vi "P3 E1 RLJ 2015640305.vi"() -> ()   [LabVIEW 2016]
doc: "Use this template to build a simple state machine design pattern. Each state executes code and determines which state to transition to."
uses:
  State.ctl
  Data.ctl
  Control 3.ctl
panel:
  in  "abortar":bool
  in  "Exit":bool
  out "Tab":T1(tab)
  in  "id":bool
  out "Boolean":bool
  out "Pict Ring":i32(ring)
  in  "ok":bool
  in  "0":bool
  in  "8":bool
  in  "9":bool
  in  "7":bool
  in  "6":bool
  in  "5":bool
  in  "4":bool
  in  "3":bool
  in  "2":bool
  in  "1":bool
  out "concatenated string 2":string
  in  "s 2":bool
  out "String 3":string
  in  "edo de cuenta":bool
  in  "deposito oc":bool
  in  "donativo":bool
  in  "pago de tiempo aire":bool
  in  "pago de tarjeta":bool
  in  "retiro":bool
  in  "SALIR":bool
  in  "ingresar":bool
  out "String":string
  in  "Numeric Control 2":dbl
  in  "abonar":bool
  in  "Numeric Control":dbl
  out "String 2":string
  out "Array 2":bool[](array[boolean])
  in  "100":bool
  in  "200":bool
  in  "300":bool
  in  "500":bool
  out "String 4":string
  in  "CDH Tepeyac":bool
  in  "CILAS":bool
  in  "ALAMPYME":bool
  in  "nicolasa":bool
  out "String 6":string
  in  "pedro":bool
  in  "juan":bool
  in  "s 3":bool
  out "concate":string
  in  "ok 2":bool
  in  "0 2":bool
  in  "8 2":bool
  in  "9 2":bool
  in  "7 2":bool
  in  "6 2":bool
  in  "5 2":bool
  in  "4 2":bool
  in  "3 2":bool
  in  "2 2":bool
  in  "1 2":bool
  out "String 7":string
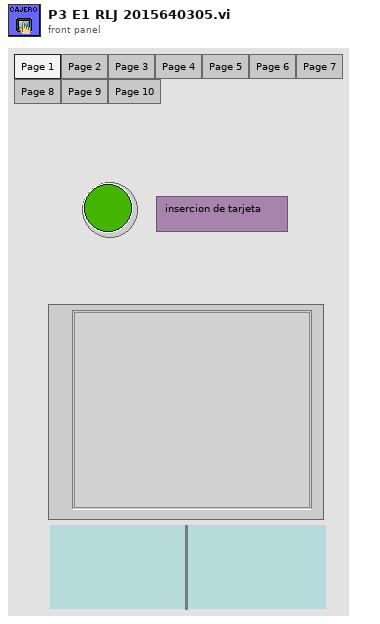
[diagram p1: front panel]
types:
  T1 = enum32{"Page 1", "Page 2", "Page 3", "Page 4", "Page 5", "Page 6", "Page 7", "Page 8", "Page 9", "Page 10"}
  T2 = typedef "Data.ctl" = cluster{"true/false":bool, "String 1":string, "saldo":dbl, "deuda":dbl, "id":bool, "pag1":bool, "seleccion":bool, "edo de cuentas":string, "cuenta error":dbl}
  T3 = typedef "State.ctl" = enum16{"Initialize", "Wait for Event", "id", "contraseña", "error", "retiro de efectivo", "pago de tarjeta", "compra de tiempo aire", "estado de cuenta", "donativo", "deposito a otra cuentas", "teclado", "menu", "abortar", "Exit"}
  T4 = typedef "Control 3.ctl" = enum32{"Page 1", "Page 2", "Page 3", "Page 4", "Page 5", "Page 6", "Page 7", "Page 8", "Page 9", "Page 10"}
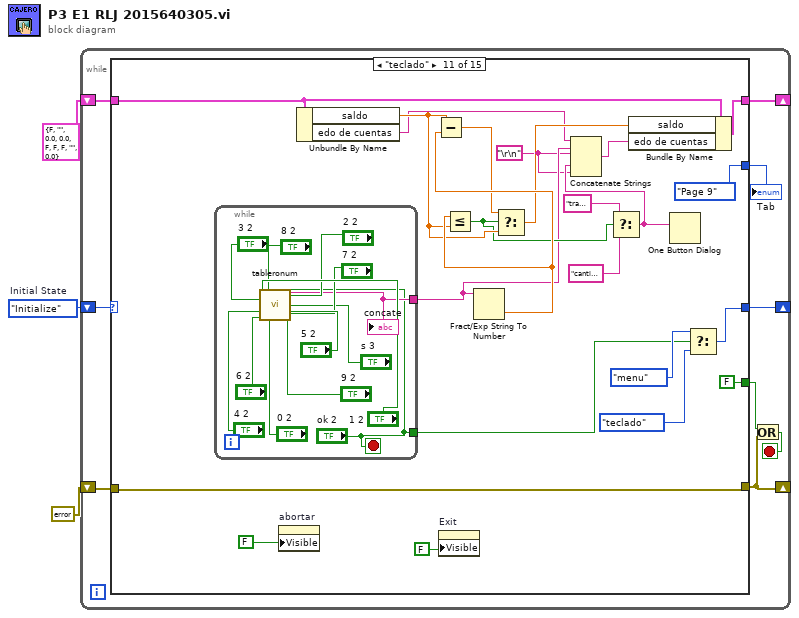
[diagram p0: block diagram]
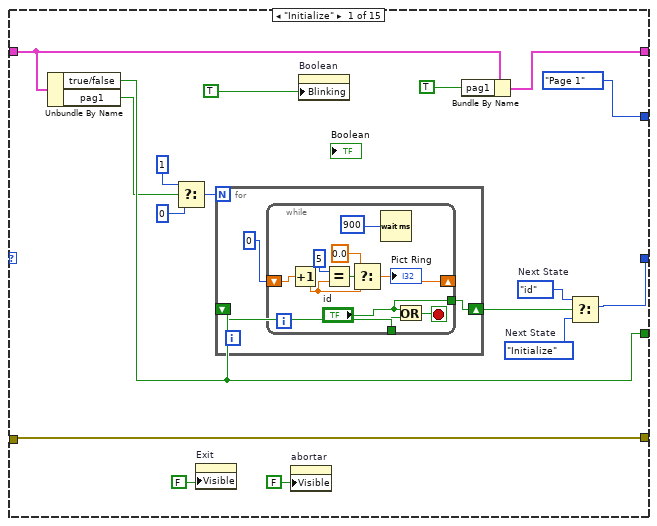
[diagram p2: hidden frame]
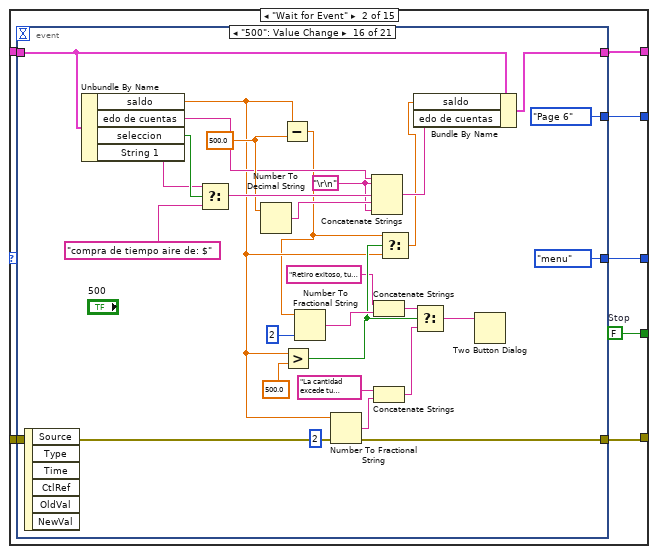
[diagram p3: hidden frame]
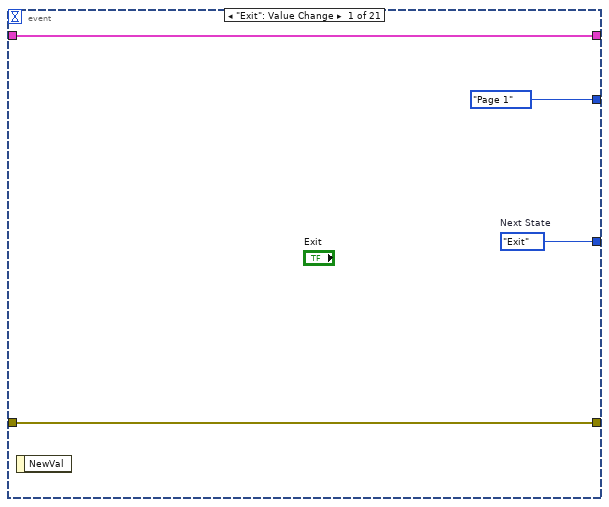
[diagram p4: hidden frame]
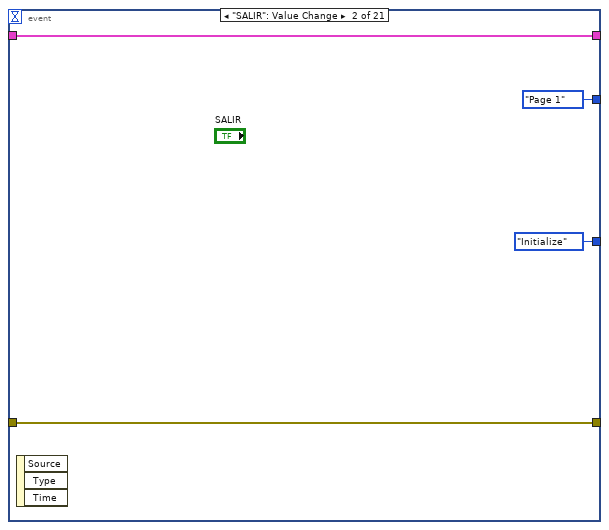
[diagram p5: hidden frame]
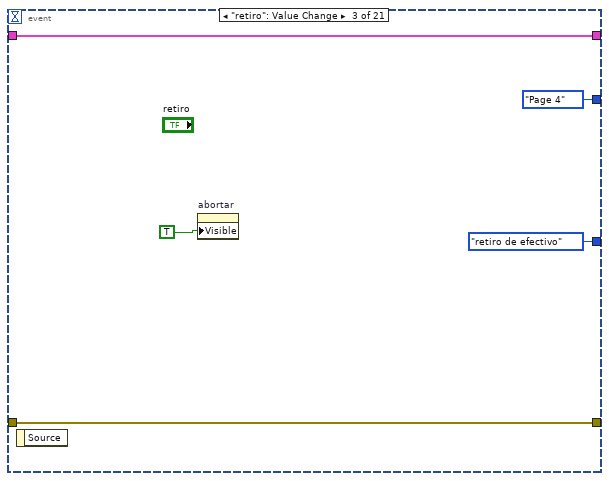
[diagram p6: hidden frame]
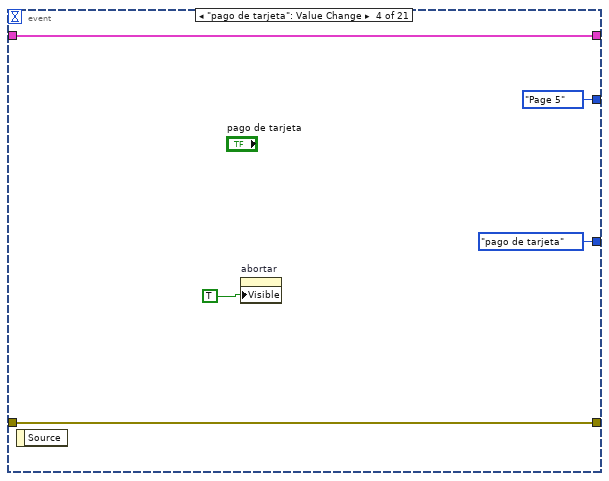
[diagram p7: hidden frame]
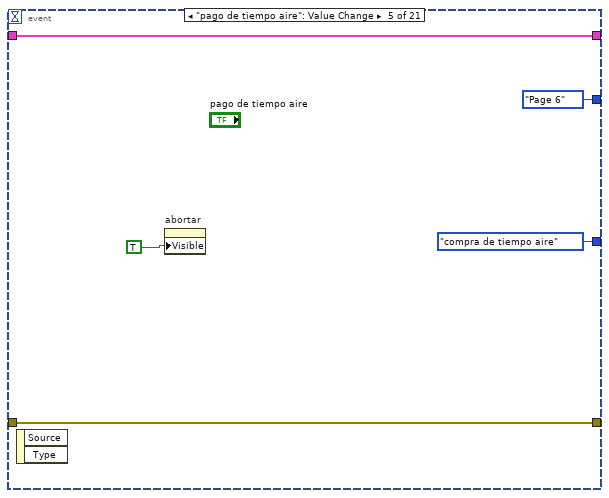
[diagram p8: hidden frame]
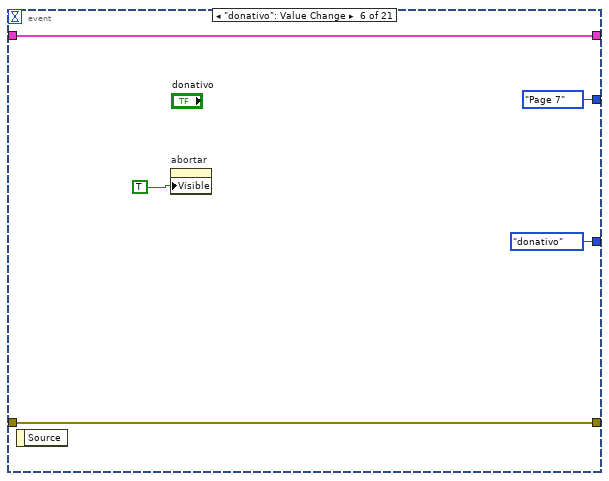
[diagram p9: hidden frame]
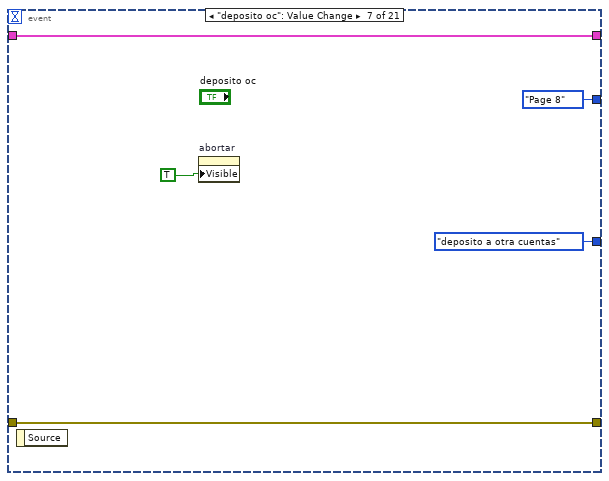
[diagram p10: hidden frame]
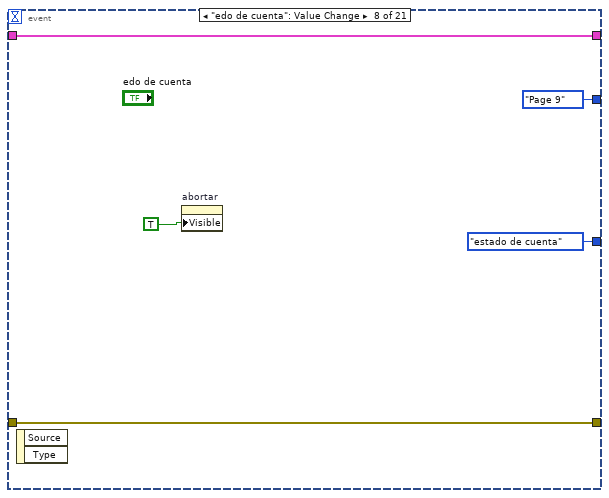
[diagram p11: hidden frame]
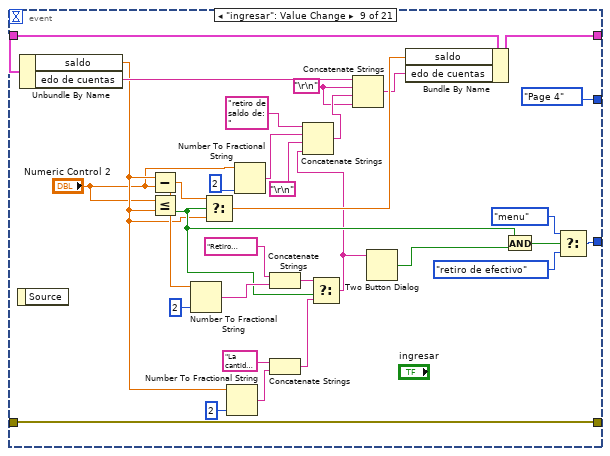
[diagram p12: hidden frame]
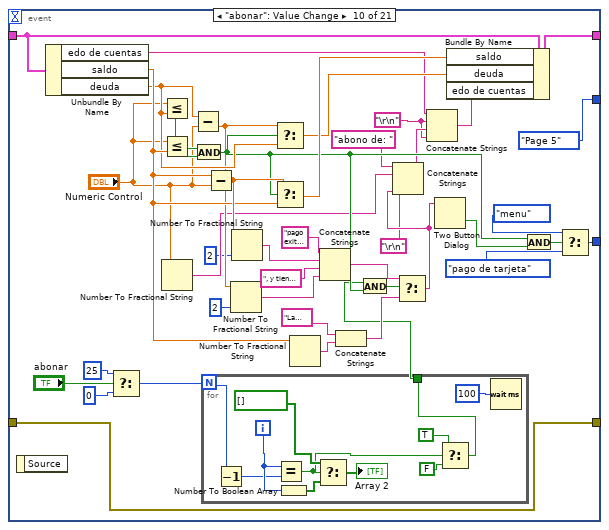
[diagram p13: hidden frame]
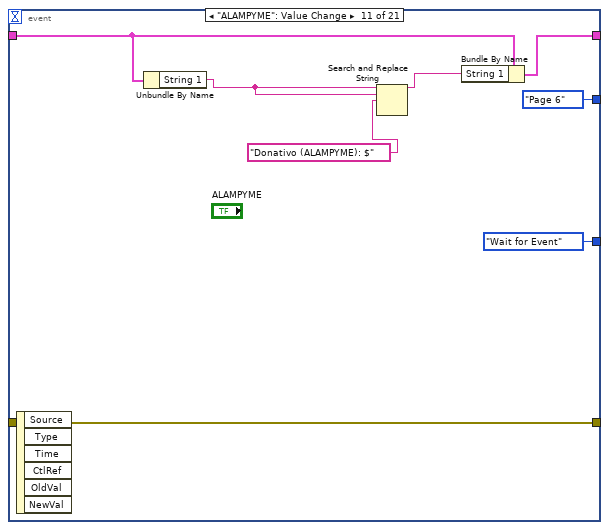
[diagram p14: hidden frame]
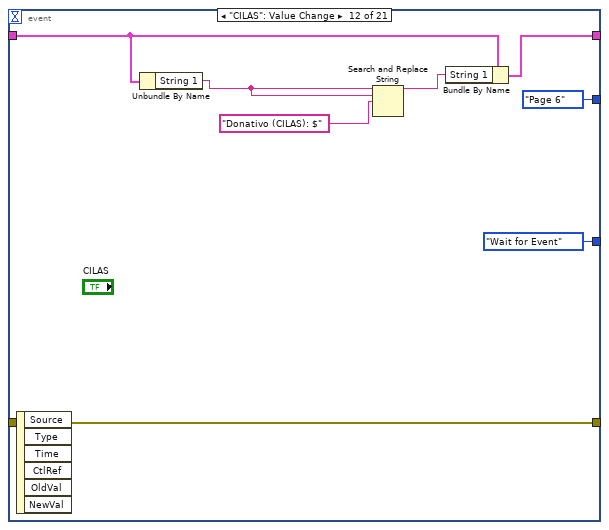
[diagram p15: hidden frame]
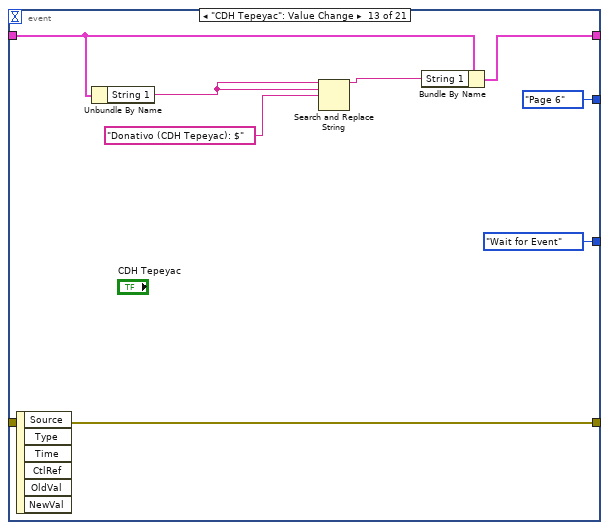
[diagram p16: hidden frame]
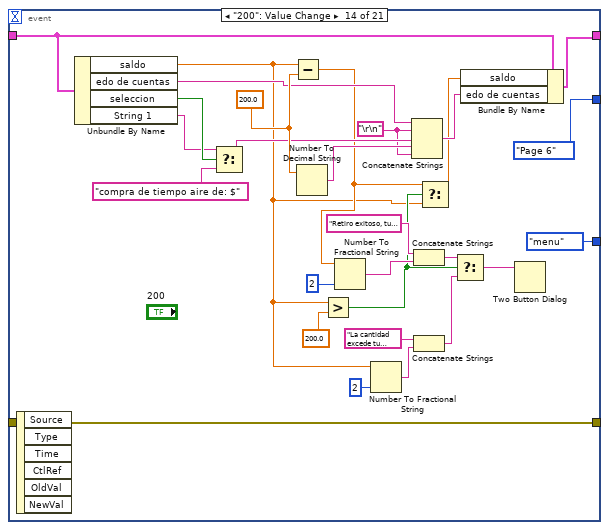
[diagram p17: hidden frame]
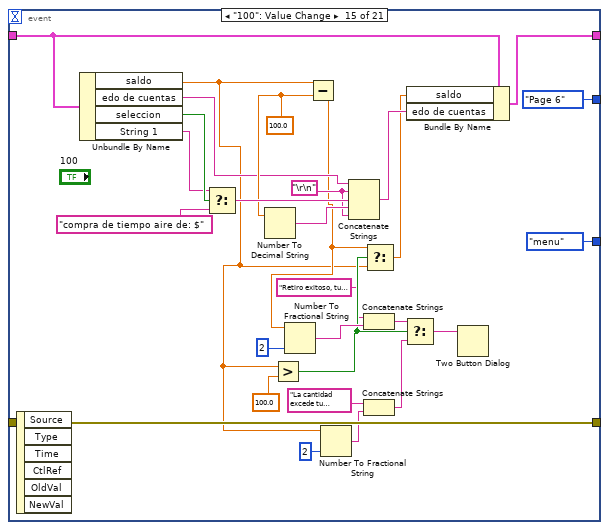
[diagram p18: hidden frame]
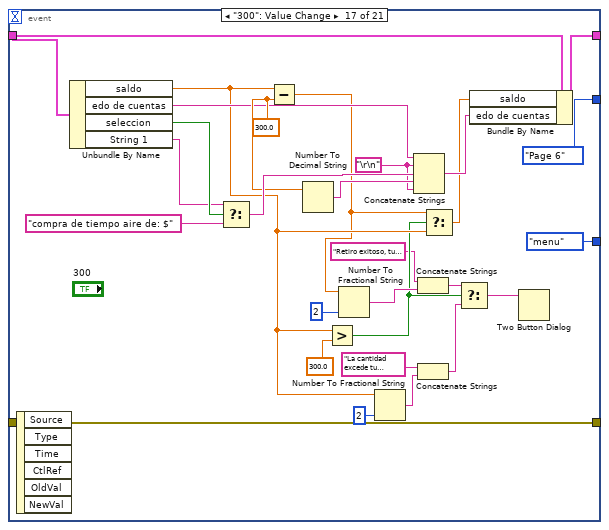
[diagram p19: hidden frame]
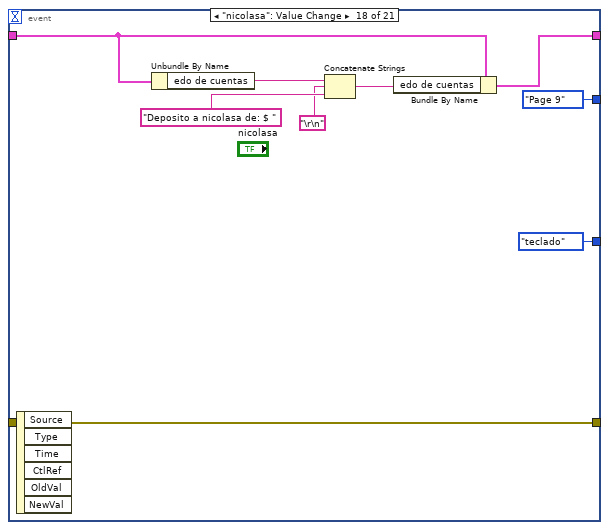
[diagram p20: hidden frame]
diagram:
  w1 = State."Initialize"  # Initial State
  n1 = while {
    shift-right: [w11] -> _
    shift-left: w1 -> [w12]
    shift-right: [w6] -> _
    shift-left: T2 {"true/false"=FALSE, "String 1"="", "saldo"=0.0, "deuda"=0.0, "id"=FALSE, "pag1"=FALSE, "seleccion"=FALSE, "edo de cuentas"="", "cuenta error"=0.0} ("Data") -> [w10]
    shift-right: [w4] -> _
    shift-left: errorcluster {"status"=FALSE, "code"=0, "source"=""} ("error constant") -> [w9]
    stop <- w8 stop-if-true
    # "Main VI State Machine"
    n2 = case shown="\"teclado\"" w12 {
      tunnel: [w28 w49 w344 w373 w393 State."Wait for Event" ("(Value Not Used)") State."Wait for Event" ("(Value Not Used)") State."Wait for Event" ("(Value Not Used)") State."Wait for Event" ("(Value Not Used)") State."Wait for Event" ("(Value Not Used)") w484 State."Wait for Event" ("(Value Not Used)") State."Wait for Event" ("(Value Not Used)") State."menu" ("(Value Not Used)") State."Initialize" ("(Value Not Used)")] -> w11
      tunnel: [w22 w48 FALSE ("Stop Loop?") FALSE ("Stop Loop?") FALSE ("Stop Loop?") FALSE ("Stop Loop?") FALSE ("Stop Loop?") FALSE ("Stop Loop?") FALSE ("Stop Loop?") FALSE ("Stop Loop?") FALSE ("Stop Loop?") FALSE ("Stop Loop?") FALSE ("Stop Loop?") FALSE ("Stop Loop?") TRUE ("Stop Loop?")] -> w5
      tunnel: w10 -> [w16 w47 w341 w371 w385 w415 w425 w435 w451 w456 w487 w505 w514 w531 w536]
      tunnel: [w15 w46 w341 w372 w384 w415 w425 w435 w450 w456 w488 w505 w522 w531 w536] -> w6
      tunnel: w9 -> [w29 w45 w349 w379 w398 w418 w429 w447 w455 w468 w491 w512 w526 w530 w535]
      tunnel: [w29 w44 w349 w379 w398 w418 w429 w447 w455 w468 w491 w512 w526 w530 w535] -> w4
      tunnel: [Control_3."Page 1" ("Tab Control") w43 Control_3."Page 2" ("Tab Control") w369 w389 Control_3."Page 3" ("Tab Control") Control_3."Page 4" ("Tab Control") Control_3."Page 5" ("Tab Control") Control_3."Page 6" ("Tab Control") Control_3."Page 8" ("Tab Control") Control_3."Page 9" ("Tab Control") Control_3."Page 10" ("Tab Control") Control_3."Page 7" ("Tab Control") Control_3."Page 3" ("Tab Control") Control_3."Page 1" ("Tab Control")] -> w7
      frame "Initialize" {
        w26 = State."Initialize"  # Next State
        w27 = State."id"  # Next State
        # "Initialize - Initialize the application."
        n3 = Unbundle By Name(w16) -> ("true/false"=w22:bool, "pag1"=w17:bool)
        n4 = Select(t=1, s=w17, f=0) -> (s? t:f=w20:i32)
        n5 = property on="Exit" class="Bool"("Visible"=FALSE) -> ()  [unwired: 2 in, 2 out]
        n6 = for {
          N: w20 -> [_]
          shift-right: [w30] -> w21
          shift-left: w22 -> [w31]
          n7 = while {
            shift-right: [w39] -> _
            shift-left: 0 -> [w41]
            tunnel: w31 -> [w34]
            tunnel: ["id"] -> w30
            stop <- w35 stop-if-true
            n8 = Increment(x=w41) -> (x+1=w36:dbl)
            n9 = Equal?(x=5, y=w36) -> (x = y?=w38:bool)
            n10 = Select(t=0.0, s=w38, f=w36) -> (s? t:f=w39:dbl)
            "Pict Ring" <- w39
            n11 = Wait (ms)(milliseconds to wait=u32 900) -> ()  [unwired: 1 out]
            n12 = Or(x="id", y=w34) -> (x .or. y?=w35:bool)
          }
        }
        n13 = property on="abortar" class="Bool"("Visible"=FALSE) -> ()  [unwired: 2 in, 2 out]
        n14 = property on="Boolean" class="Bool (strict)"("Blinking"=TRUE) -> ()  [unwired: 2 in, 2 out]
        n15 = Bundle By Name(cluster=w16, "pag1"=TRUE ("corrimiento")) -> (w15:T2)
        n16 = Select(t=w27, s=w21, f=w26) -> (s? t:f=w28:T3)
      }
      frame "Wait for Event" {
        w48 = FALSE  # Stop
        n17 = event shown="[15] \"500\": Value Change" {
          selector: _ -> [_ _ _ _ _ _ _ _ _ _ _ _ _ _ _ _ _ _ _ _ _]
          dyn-events: _ -> [_ _ _ _ _ _ _ _ _ _ _ _ _ _ _ _ _ _ _ _ _]
          timeout: _ -> [_ _ _ _ _ _ _ _ _ _ _ _ _ _ _ _ _ _ _ _ _]
          tunnel: [w53 State."Initialize" ("f") State."retiro de efectivo" ("f") State."pago de tarjeta" ("f") State."compra de tiempo aire" ("f") State."donativo" ("f") State."deposito a otra cuentas" ("f") State."estado de cuenta" ("f") w108 w145 State."Wait for Event" ("f") State."Wait for Event" ("f") State."Wait for Event" ("f") State."menu" ("f") State."menu" ("f") State."menu" ("f") State."menu" ("f") State."teclado" ("f") State."teclado" ("f") State."teclado" ("f") State."menu" ("f")] -> w49
          tunnel: w47 -> [w52 w57 w62 w67 w72 w77 w82 w87 w104 w147 w176 w181 w189 w221 w249 w277 w305 w312 w322 w330 w339]
          tunnel: [w52 w57 w62 w67 w72 w77 w82 w87 w101 w146 w179 w187 w195 w220 w248 w276 w304 w311 w323 w329 w339] -> w46
          tunnel: w45 -> [w51 w56 w61 w66 w71 w76 w81 w86 w118 w161 w180 w188 w196 w224 w252 w280 w308 w317 w326 w335 w338]
          tunnel: [w51 w56 w61 w66 w71 w76 w81 w86 w118 w161 w180 w188 w196 w224 w252 w280 w308 w317 w326 w335 w338] -> w44
          tunnel: [Control_3."Page 1" ("Tab Control") Control_3."Page 1" ("Tab Control") Control_3."Page 4" ("Tab Control") Control_3."Page 5" ("Tab Control") Control_3."Page 6" ("Tab Control") Control_3."Page 7" ("Tab Control") Control_3."Page 8" ("Tab Control") Control_3."Page 9" ("Tab Control") Control_3."Page 4" ("Tab Control") Control_3."Page 5" ("Tab Control") Control_3."Page 6" ("Tab Control") Control_3."Page 6" ("Tab Control") Control_3."Page 6" ("Tab Control") Control_3."Page 6" ("Tab Control") Control_3."Page 6" ("Tab Control") Control_3."Page 6" ("Tab Control") Control_3."Page 6" ("Tab Control") Control_3."Page 9" ("Tab Control") Control_3."Page 9" ("Tab Control") Control_3."Page 9" ("Tab Control") Control_3."Page 3" ("Tab Control")] -> w43
          event "Exit": Value Change {
            w53 = State."Exit"  # Next State
            n18 = event-data() -> ()  [unwired: 1 in, 1 out]
          }
          event "SALIR": Value Change {
            n19 = event-data() -> ()  [unwired: 1 in, 3 out]
          }
          event "retiro": Value Change {
            n20 = event-data() -> ()  [unwired: 1 in, 1 out]
            n21 = property on="abortar" class="Bool"("Visible"=TRUE) -> ()  [unwired: 2 in, 2 out]
          }
          event "pago de tarjeta": Value Change {
            n22 = event-data() -> ()  [unwired: 1 in, 1 out]
            n23 = property on="abortar" class="Bool"("Visible"=TRUE) -> ()  [unwired: 2 in, 2 out]
          }
          event "pago de tiempo aire": Value Change {
            n24 = event-data() -> ()  [unwired: 1 in, 2 out]
            n25 = property on="abortar" class="Bool"("Visible"=TRUE) -> ()  [unwired: 2 in, 2 out]
          }
          event "donativo": Value Change {
            n26 = event-data() -> ()  [unwired: 1 in, 1 out]
            n27 = property on="abortar" class="Bool"("Visible"=TRUE) -> ()  [unwired: 2 in, 2 out]
          }
          event "deposito oc": Value Change {
            n28 = event-data() -> ()  [unwired: 1 in, 1 out]
            n29 = property on="abortar" class="Bool"("Visible"=TRUE) -> ()  [unwired: 2 in, 2 out]
          }
          event "edo de cuenta": Value Change {
            n30 = event-data() -> ()  [unwired: 1 in, 2 out]
            n31 = property on="abortar" class="Bool"("Visible"=TRUE) -> ()  [unwired: 2 in, 2 out]
          }
          event "ingresar": Value Change {
            w91 = "\r\n"
            n32 = event-data() -> ()  [unwired: 1 in, 1 out]
            n33 = Unbundle By Name(w104) -> ("saldo"=w93:dbl, "edo de cuentas"=w100:string)
            n34 = Subtract(x=w93, y="Numeric Control 2") -> (x-y=w117:dbl)
            n35 = Less Or Equal?(x="Numeric Control 2", y=w93) -> (x <= y?=w110:bool)
            n36 = Number To Fractional String(number=w117, precision (6)=i16 2) -> (F-format string=w116:string)  [unwired: 2 in]
            n37 = Select(t=w117, s=w110, f=w93) -> (s? t:f=w103:dbl)
            n38 = Number To Fractional String(number=w93, precision (6)=i16 2) -> (F-format string=w113:string)  [unwired: 2 in]
            n39 = Number To Fractional String(number="Numeric Control 2", precision (6)=i16 2) -> (F-format string=w98:string)  [unwired: 2 in]
            n40 = Concatenate Strings("Retiro exitoso, tu saldo actual es de: \n" ("string"), w116) -> (w115:string)
            n41 = Concatenate Strings("La cantidad excede tu credito, el cual es de: \n" ("string"), w113) -> (w112:string)
            n42 = Select(t=w115, s=w110, f=w112) -> (s? t:f=w95:string)
            n43 = Concatenate Strings("retiro de saldo de: " ("string"), w98, "\r\n", w95) -> (w96:string)
            n44 = Concatenate Strings(w100, w91, w96, w91) -> (w99:string)
            n45 = Two Button Dialog(message=w95) -> (T button?=w111:bool)  [unwired: 2 in]
            n46 = Bundle By Name(cluster=w104, "saldo"=w103, "edo de cuentas"=w99) -> (w101:T2)
            n47 = And(x=w110, y=w111) -> (x .and. y?=w109:bool)
            n48 = Select(t=State."menu" ("Next State"), s=w109, f=State."retiro de efectivo") -> (s? t:f=w108:T3)
          }
          event "abonar": Value Change {
            w123 = "\r\n"
            n49 = event-data() -> ()  [unwired: 1 in, 1 out]
            n50 = Unbundle By Name(w147) -> ("edo de cuentas"=w130:string, "saldo"=w154:dbl, "deuda"=w141:dbl)
            n51 = Select(t=25, s="abonar", f=0) -> (s? t:f=w137:i32)
            n52 = Less Or Equal?(x="Numeric Control", y=w141) -> (x <= y?=w144:bool)
            n53 = Less Or Equal?(x="Numeric Control", y=w154) -> (x <= y?=w143:bool)
            n54 = Number To Fractional String(number="Numeric Control") -> (F-format string=w127:string)  [unwired: 3 in]
            n55 = Subtract(x=w141, y="Numeric Control") -> (x-y=w132:dbl)
            n56 = And(x=w144, y=w143) -> (x .and. y?=w136:bool)
            n57 = for {
              N: w137 -> [w170]
              tunnel: [w162] -> w134
              i -> [w171]
              n58 = Decrement(x=w170) -> (x-1=w169:i32)
              n59 = Equal?(x=w171, y=w169) -> (x = y?=w165:bool)
              n60 = Number To Boolean Array(number=w171) -> (Boolean array=w168:bool[])
              n61 = Select(t=bool[] [], s=w165, f=w168) -> (s? t:f=→"Array 2":bool[])
              n62 = Select(t=TRUE, s=w165, f=FALSE) -> (s? t:f=w162:bool)
              n63 = Wait (ms)(milliseconds to wait=u32 100) -> ()  [unwired: 1 out]
            }
            n64 = Subtract(x=w154, y="Numeric Control") -> (x-y=w160:dbl)
            n65 = Number To Fractional String(number=w132, precision (6)=i16 2) -> (F-format string=w122:string)  [unwired: 2 in]
            n66 = Number To Fractional String(number=w160, precision (6)=i16 2) -> (F-format string=w159:string)  [unwired: 2 in]
            n67 = Select(t=w132, s=w136, f=w141) -> (s? t:f=w142:dbl)
            n68 = Select(t=w160, s=w136, f=w154) -> (s? t:f=w148:dbl)
            n69 = Number To Fractional String(number=w154) -> (F-format string=w156:string)  [unwired: 3 in]
            n70 = Concatenate Strings("pago exitoso, tu saldo actual es de: \n" ("string"), w159, ", y tienes un adeudo de: " ("string"), w122) -> (w158:string)
            n71 = Concatenate Strings("La cantidad excede tu credito, el cual es de: \n" ("string"), w156) -> (w155:string)
            n72 = And(x=w134, y=w136) -> (x .and. y?=w133:bool)
            n73 = Select(t=w158, s=w133, f=w155) -> (s? t:f=w125:string)
            n74 = Concatenate Strings("abono de: " ("string"), w127, "\r\n", w125) -> (w126:string)
            n75 = Concatenate Strings(w130, w123, w126, w123) -> (w131:string)
            n76 = Two Button Dialog(message=w125) -> (T button?=w153:bool)  [unwired: 2 in]
            n77 = Bundle By Name(cluster=w147, "saldo"=w148, "deuda"=w142, "edo de cuentas"=w131) -> (w146:T2)
            n78 = And(x=w136, y=w153) -> (x .and. y?=w152:bool)
            n79 = Select(t=State."menu" ("Next State"), s=w152, f=State."pago de tarjeta") -> (s? t:f=w145:T3)
          }
          event "ALAMPYME": Value Change {
            n80 = event-data() -> ()  [unwired: 1 in, 6 out]
            n81 = Unbundle By Name(w176) -> ("String 1"=w175:string)
            n82 = Search and Replace String(input string=w175, search string=w175, replace string="Donativo (ALAMPYME): $" ("String <Replace Me>")) -> (result string=w173:string)  [unwired: 5 in, 3 out]
            n83 = Bundle By Name(cluster=w176, "String 1"=w173) -> (w179:T2)
          }
          event "CILAS": Value Change {
            n84 = event-data() -> ()  [unwired: 1 in, 6 out]
            n85 = Unbundle By Name(w181) -> ("String 1"=w184:string)
            n86 = Search and Replace String(input string=w184, search string=w184, replace string="Donativo (CILAS): $" ("String <Replace Me>")) -> (result string=w183:string)  [unwired: 5 in, 3 out]
            n87 = Bundle By Name(cluster=w181, "String 1"=w183) -> (w187:T2)
          }
          event "CDH Tepeyac": Value Change {
            n88 = event-data() -> ()  [unwired: 1 in, 6 out]
            n89 = Unbundle By Name(w189) -> ("String 1"=w192:string)
            n90 = Search and Replace String(input string=w192, search string=w192, replace string="Donativo (CDH Tepeyac): $" ("String <Replace Me>")) -> (result string=w190:string)  [unwired: 5 in, 3 out]
            n91 = Bundle By Name(cluster=w189, "String 1"=w190) -> (w195:T2)
          }
          event "200": Value Change {
            w211 = "\r\n"
            w219 = 200.0 ("y")
            n92 = event-data() -> ()  [unwired: 1 in, 6 out]
            n93 = Unbundle By Name(w221) -> ("saldo"=w198:dbl, "edo de cuentas"=w212:string, "seleccion"=w217:bool, "String 1"=w213:string)
            n94 = Select(t=w213, s=w217, f="compra de tiempo aire de: $") -> (s? t:f=w215:string)
            n95 = Subtract(x=w198, y=w219) -> (x-y=w199:dbl)
            n96 = Number To Decimal String(number=w219) -> (decimal integer string=w214:string)  [unwired: 1 in]
            n97 = Greater?(x=w198, y=200.0) -> (0:w200:bool)
            n98 = Number To Fractional String(number=w199, precision (6)=i16 2) -> (F-format string=w210:string)  [unwired: 2 in]
            n99 = Number To Fractional String(number=w198, precision (6)=i16 2) -> (F-format string=w207:string)  [unwired: 2 in]
            n100 = Concatenate Strings(w212, w211, w215, w214, w211) -> (w218:string)
            n101 = Concatenate Strings("Retiro exitoso, tu saldo actual es de: \n" ("string"), w210) -> (w209:string)
            n102 = Concatenate Strings("La cantidad excede tu credito, el cual es de: \n" ("string"), w207) -> (w206:string)
            n103 = Select(t=w199, s=w200, f=w198) -> (s? t:f=w197:dbl)
            n104 = Select(t=w209, s=w200, f=w206) -> (s? t:f=w203:string)
            n105 = Bundle By Name(cluster=w221, "saldo"=w197, "edo de cuentas"=w218) -> (w220:T2)
            n106 = Two Button Dialog(message=w203) -> ()  [unwired: 2 in, 1 out]
          }
          event "100": Value Change {
            w239 = "\r\n"
            w243 = 100.0 ("y")
            n107 = event-data() -> ()  [unwired: 1 in, 6 out]
            n108 = Unbundle By Name(w249) -> ("saldo"=w226:dbl, "edo de cuentas"=w240:string, "seleccion"=w242:bool, "String 1"=w241:string)
            n109 = Select(t=w241, s=w242, f="compra de tiempo aire de: $") -> (s? t:f=w246:string)
            n110 = Number To Decimal String(number=w243) -> (decimal integer string=w245:string)  [unwired: 1 in]
            n111 = Greater?(x=w226, y=100.0) -> (0:w229:bool)
            n112 = Subtract(x=w226, y=w243) -> (x-y=w227:dbl)
            n113 = Number To Fractional String(number=w227, precision (6)=i16 2) -> (F-format string=w238:string)  [unwired: 2 in]
            n114 = Number To Fractional String(number=w226, precision (6)=i16 2) -> (F-format string=w235:string)  [unwired: 2 in]
            n115 = Concatenate Strings(w240, w239, w246, w245, w239) -> (w244:string)
            n116 = Concatenate Strings("Retiro exitoso, tu saldo actual es de: \n" ("string"), w238) -> (w237:string)
            n117 = Concatenate Strings("La cantidad excede tu credito, el cual es de: \n" ("string"), w235) -> (w234:string)
            n118 = Select(t=w227, s=w229, f=w226) -> (s? t:f=w225:dbl)
            n119 = Select(t=w237, s=w229, f=w234) -> (s? t:f=w232:string)
            n120 = Bundle By Name(cluster=w249, "saldo"=w225, "edo de cuentas"=w244) -> (w248:T2)
            n121 = Two Button Dialog(message=w232) -> ()  [unwired: 2 in, 1 out]
          }
          event "500": Value Change {
            w270 = 500.0 ("y")
            w267 = "\r\n"
            n122 = event-data() -> ()  [unwired: 1 in, 6 out]
            n123 = Unbundle By Name(w277) -> ("saldo"=w256:dbl, "edo de cuentas"=w268:string, "seleccion"=w271:bool, "String 1"=w269:string)
            n124 = Select(t=w269, s=w271, f="compra de tiempo aire de: $") -> (s? t:f=w274:string)
            n125 = Number To Decimal String(number=w270) -> (decimal integer string=w273:string)  [unwired: 1 in]
            n126 = Subtract(x=w256, y=w270) -> (x-y=w255:dbl)
            n127 = Greater?(x=w256, y=500.0) -> (0:w257:bool)
            n128 = Number To Fractional String(number=w255, precision (6)=i16 2) -> (F-format string=w266:string)  [unwired: 2 in]
            n129 = Number To Fractional String(number=w256, precision (6)=i16 2) -> (F-format string=w263:string)  [unwired: 2 in]
            n130 = Concatenate Strings(w268, w267, w274, w273, w267) -> (w272:string)
            n131 = Concatenate Strings("Retiro exitoso, tu saldo actual es de: \n" ("string"), w266) -> (w265:string)
            n132 = Concatenate Strings("La cantidad excede tu credito, el cual es de: \n" ("string"), w263) -> (w262:string)
            n133 = Select(t=w255, s=w257, f=w256) -> (s? t:f=w254:dbl)
            n134 = Bundle By Name(cluster=w277, "saldo"=w254, "edo de cuentas"=w272) -> (w276:T2)
            n135 = Select(t=w265, s=w257, f=w262) -> (s? t:f=w260:string)
            n136 = Two Button Dialog(message=w260) -> ()  [unwired: 2 in, 1 out]
          }
          event "300": Value Change {
            w295 = "\r\n"
            w300 = 300.0 ("y")
            n137 = event-data() -> ()  [unwired: 1 in, 6 out]
            n138 = Unbundle By Name(w305) -> ("saldo"=w285:dbl, "edo de cuentas"=w296:string, "seleccion"=w298:bool, "String 1"=w297:string)
            n139 = Select(t=w297, s=w298, f="compra de tiempo aire de: $") -> (s? t:f=w302:string)
            n140 = Subtract(x=w285, y=w300) -> (x-y=w283:dbl)
            n141 = Number To Decimal String(number=w300) -> (decimal integer string=w301:string)  [unwired: 1 in]
            n142 = Greater?(x=w285, y=300.0) -> (0:w284:bool)
            n143 = Number To Fractional String(number=w283, precision (6)=i16 2) -> (F-format string=w294:string)  [unwired: 2 in]
            n144 = Number To Fractional String(number=w285, precision (6)=i16 2) -> (F-format string=w291:string)  [unwired: 2 in]
            n145 = Concatenate Strings(w296, w295, w302, w301, w295) -> (w299:string)
            n146 = Concatenate Strings("Retiro exitoso, tu saldo actual es de: \n" ("string"), w294) -> (w293:string)
            n147 = Concatenate Strings("La cantidad excede tu credito, el cual es de: \n" ("string"), w291) -> (w290:string)
            n148 = Select(t=w283, s=w284, f=w285) -> (s? t:f=w282:dbl)
            n149 = Select(t=w293, s=w284, f=w290) -> (s? t:f=w288:string)
            n150 = Bundle By Name(cluster=w305, "saldo"=w282, "edo de cuentas"=w299) -> (w304:T2)
            n151 = Two Button Dialog(message=w288) -> ()  [unwired: 2 in, 1 out]
          }
          event "nicolasa": Value Change {
            n152 = event-data() -> ()  [unwired: 1 in, 6 out]
            n153 = Unbundle By Name(w312) -> ("edo de cuentas"=w313:string)
            n154 = Concatenate Strings(w313, "\r\n", "Deposito a nicolasa de: $ " ("string")) -> (w314:string)
            n155 = Bundle By Name(cluster=w312, "edo de cuentas"=w314) -> (w311:T2)
          }
          event "juan": Value Change {
            n156 = event-data() -> ()  [unwired: 1 in, 6 out]
            n157 = Unbundle By Name(w322) -> ("edo de cuentas"=w321:string)
            n158 = Concatenate Strings(w321, "\r\n", "Deposito a juan de: $ " ("string")) -> (w320:string)
            n159 = Bundle By Name(cluster=w322, "edo de cuentas"=w320) -> (w323:T2)
          }
          event "pedro": Value Change {
            n160 = event-data() -> ()  [unwired: 1 in, 6 out]
            n161 = Unbundle By Name(w330) -> ("edo de cuentas"=w331:string)
            n162 = Concatenate Strings(w331, "\r\n", "Deposito a pedro de: $ " ("string")) -> (w332:string)
            n163 = Bundle By Name(cluster=w330, "edo de cuentas"=w332) -> (w329:T2)
          }
          event "abortar": Value Change {
            n164 = event-data() -> ()  [unwired: 1 in, 2 out]
          }
        }
      }
      frame "contraseña" {
        w345 = State."error"  # Next State
        w346 = State."menu"  # Next State
        n165 = while {
          tunnel: [w352] -> w342
          stop <- "ok" stop-if-true
          n166 = call "tableronum.vi"("1"="1", "8"="8", "OK"="ok", "3"="3", "2"="2", "s 2"="s 2", "4"="4", "5"="5", "6"="6", "0"="0", "7"="7", "9"="9") -> ("concatenated string"=w352:string)  [unwired: 3 in]
          "concatenated string 2" <- w352
        }
        n167 = Unbundle By Name(w341) -> ()  [unwired: 1 out]
        n168 = Equal?(x=w342, y="1393") -> (x = y?=w343:bool)
        n169 = Select(t=w346, s=w343, f=w345) -> (s? t:f=w344:T3)
      }
      frame "error" {
        n170 = Unbundle By Name(w371) -> ("cuenta error"=w370:dbl)
        n171 = Increment(x=w370) -> (x+1=w377:dbl)
        n172 = Equal?(x=w377, y=3.0) -> (x = y?=w366:bool)
        n173 = Bundle By Name(cluster=w371, "cuenta error"=w377, "true/false"=w366) -> (w372:T2)
        n174 = Select(t="Cancelación de sesión" ("message"), s=w366, f="error" ("message")) -> (s? t:f=w363:string)
        n175 = One Button Dialog(message=w363) -> ()  [unwired: 1 in, 1 out]
        n176 = Select(t=Control_3."Page 1" ("Tab Control"), s=w366, f=Control_3."Page 2" ("Tab Control")) -> (s? t:f=w369:T4)
        n177 = Select(t=State."Initialize" ("(Value Not Used)"), s=w366, f=State."contraseña" ("(Value Not Used)")) -> (s? t:f=w373:T3)
      }
      frame "id" {
        w394 = State."Initialize"  # Initial State
        w395 = State."contraseña"  # Initial State
        # "User State 1 - Replace this state with functionality for your own application."
        n178 = Random Number (0-1)() -> (number: 0 to 1=w386:dbl)
        n179 = Random Number (0-1)() -> (number: 0 to 1=w387:dbl)
        n180 = expression code="6000-(1000*x)"(w386) -> (w383:dbl)
        n181 = expression code="10000-(6000*x)"(w387) -> (w381:dbl)
        n182 = To Quad Integer(1:w383) -> (0:w382:i64)
        n183 = To Quad Integer(1:w381) -> (0:w380:i64)
        n184 = Bundle By Name(cluster=w385, "saldo"=w382, "deuda"=w380) -> (w384:T2)
        n185 = Two Button Dialog(message="es usted Ramirez lopez jesus alberto\ncon numero de boleta 2015640305" ("Running User State 1"), 1:"no" ("F button name (\"Cancel\")"), 2:"si" ("T button name (\"OK\")")) -> (T button?=w391:bool)
        n186 = Select(t=w395, s=w391, f=w394) -> (s? t:f=w393:T3)
        n187 = Select(t=Control_3."Page 2" ("Tab Control"), s=w391, f=Control_3."Page 1" ("Tab Control")) -> (s? t:f=w389:T4)
      }
      frame "menu" {
        n188 = Unbundle By Name(w415) -> ("saldo"=w408:dbl, "deuda"=w402:dbl)
        n189 = property on="Exit" class="Bool"("Visible"=TRUE) -> ()  [unwired: 2 in, 2 out]
        n190 = property on="abortar" class="Bool"("Visible"=FALSE) -> ()  [unwired: 2 in, 2 out]
        n191 = Number To Fractional String(number=w402, precision (6)=i16 2) -> (F-format string=w406:string)  [unwired: 2 in]
        n192 = Number To Fractional String(number=w408, precision (6)=i16 2) -> (F-format string=w413:string)  [unwired: 2 in]
        n193 = Concatenate Strings("TU SALDO ES DE:   " ("message"), w413) -> (w410:string)
        n194 = Concatenate Strings("TU DEUDA ES DE:   " ("message"), w406) -> (w409:string)
        n195 = Concatenate Strings(w410, "\r\n", w409) -> (→"String 3":string)
      }
      frame "retiro de efectivo" {
        n196 = Unbundle By Name(w425) -> ("saldo"=w420:dbl)
        n197 = Number To Fractional String(number=w420, precision (6)=i16 2) -> (F-format string=w424:string)  [unwired: 2 in]
        n198 = Concatenate Strings("RETIRO DE EFECTIVO:    \n tu credito es de: " ("string"), w424, "\nIngresa el valor a retirar" ("string")) -> (→"String":string)
      }
      frame "pago de tarjeta" {
        n199 = Unbundle By Name(w435) -> ("saldo"=w440:dbl)
        n200 = Unbundle By Name(w435) -> ("deuda"=w436:dbl)
        n201 = Number To Fractional String(number=w440, precision (6)=i16 2) -> (F-format string=w443:string)  [unwired: 2 in]
        n202 = Number To Fractional String(number=w436, precision (6)=i16 2) -> (F-format string=w439:string)  [unwired: 2 in]
        n203 = Concatenate Strings("PAGO DE TARJETA:    \n tu credito es de: " ("string"), w443, "\nIngresa el valor a retirar" ("string")) -> (w434:string)
        n204 = Concatenate Strings("\nsu adeudo de tarjeta de credito es de: " ("string"), w439, "\nIngresa el valor a abonar" ("string")) -> (w433:string)
        n205 = Concatenate Strings(w434, w433) -> (→"String 2":string)
      }
      frame "compra de tiempo aire" {
        n206 = Bundle By Name(cluster=w451, "String 1"="COMPRA DE TIEMPO AIRE\nselecciona el valor de tu recarga" ("String <Replace Me>"), "seleccion"=FALSE) -> (w450:T2)
      }
      frame "deposito a otra cuentas" {
        w457 = "\r\n"
        n207 = Unbundle By Name(w456) -> ("saldo"=w463:dbl)
        n208 = Number To Fractional String(number=w463, precision (6)=i16 2) -> (F-format string=w460:string)  [unwired: 2 in]
        n209 = Concatenate Strings("DEPOSITO A OTRAS CUENTAS" ("string"), w457, "Tu saldo es de: " ("string"), w457, w460, w457, "Selecciona la persona a la que realizaras el deposito:") -> (→"String 6":string)
      }
      frame "teclado" {
        w472 = "\r\n"
        n210 = while {
          tunnel: [w494] -> w474
          tunnel: ["ok 2"] -> w483
          stop <- "ok 2" stop-if-true
          n211 = call "tableronum.vi"("1"="1 2", "8"="8 2", "OK"="ok 2", "3"="3 2", "2"="2 2", "s 2"="s 3", "4"="4 2", "5"="5 2", "6"="6 2", "0"="0 2", "7"="7 2", "9"="9 2") -> ("concatenated string"=w494:string)  [unwired: 3 in]
          "concate" <- w494
        }
        n212 = property on="abortar" class="Bool"("Visible"=FALSE) -> ()  [unwired: 2 in, 2 out]
        n213 = Unbundle By Name(w487) -> ("saldo"=w479:dbl, "edo de cuentas"=w475:string)
        n214 = property on="Exit" class="Bool"("Visible"=FALSE) -> ()  [unwired: 2 in, 2 out]
        n215 = Fract/Exp String To Number(string=w474) -> (number=w482:dbl)  [unwired: 3 in, 1 out]
        n216 = Subtract(x=w479, y=w482) -> (x-y=w480:dbl)
        n217 = Less Or Equal?(x=w482, y=w479) -> (x <= y?=w478:bool)
        n218 = Select(t=w480, s=w478, f=w479) -> (s? t:f=w481:dbl)
        n219 = Select(t="transaccion exitosa", s=w478, f="cantidad incorrecta") -> (s? t:f=w473:string)
        n220 = Concatenate Strings(w475, w474, w472, w473, w472) -> (w471:string)
        n221 = Bundle By Name(cluster=w487, "saldo"=w481, "edo de cuentas"=w471) -> (w488:T2)
        n222 = One Button Dialog(message=w473) -> ()  [unwired: 1 in, 1 out]
        n223 = Select(t=State."menu" ("(Value Not Used)"), s=w483, f=State."teclado" ("(Value Not Used)")) -> (s? t:f=w484:T3)
      }
      frame "estado de cuenta" {
        n224 = Unbundle By Name(w505) -> ("edo de cuentas"=w506:string)
        n225 = Concatenate Strings("ESTADO DE CUENTA" ("string"), w506) -> (→"String 7":string)
      }
      frame "donativo" {
        w517 = "\r\n"
        w516 = "DONATIVO\nselecciona la asociacion a la que quieras donar" ("String <Replace Me>")
        n226 = Unbundle By Name(w514) -> ("saldo"=w513:dbl)
        n227 = Number To Fractional String(number=w513, precision (6)=i16 2) -> (F-format string=w518:string)  [unwired: 2 in]
        n228 = Bundle By Name(cluster=w514, "String 1"=w516, "seleccion"=TRUE) -> (w522:T2)
        n229 = Concatenate Strings(w516, w517, "Tu saldo es de: " ("string"), w517, w518, w517) -> (→"String 4":string)
      }
      frame "abortar" {
      }
      frame "Exit" {
      }
    }
    "Tab" <- w7
    n230 = Or(x=w5, y=w4) -> (x .or. y?=w8:bool)
  }
